vi "Convert 9 to g for SSD comparision.vi"(10 "String":string) -> (2 "concatenated string":string)   [LabVIEW 2016, in "Centauro.lvlib"]
uses:
  Projects/Centauro.lvlib
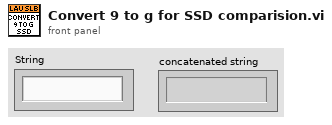
[diagram p1: front panel]
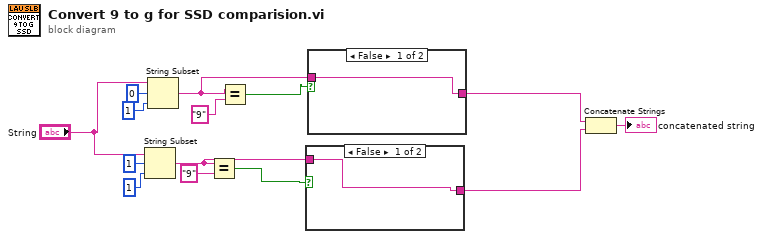
[diagram p0: block diagram]
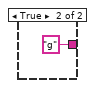
[diagram p2: hidden frame]
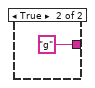
[diagram p3: hidden frame]
diagram:
  n1 = String Subset(string="String", offset (0)=1, length (rest)=1 ("length (rest)")) -> (substring=w2:string)
  n2 = String Subset(string="String", offset (0)=0, length (rest)=1 ("length (rest)")) -> (substring=w3:string)
  n3 = Equal?(x=w2, y="9") -> (x = y?=w7:bool)
  n4 = Equal?(x=w3, y="9") -> (x = y?=w6:bool)
  n5 = case shown="False" w7 {
    tunnel: [w15 "g" ("string")] -> w4
    tunnel: w2 -> [w15 _]
    frame False {
    }
    frame True {
    }
  }
  n6 = case shown="False" w6 {
    tunnel: [w17 "g" ("string")] -> w5
    tunnel: w3 -> [w17 _]
    frame False {
    }
    frame True {
    }
  }
  n7 = Concatenate Strings(w5, w4) -> (→"concatenated string":string)
